vi "Auto Move Straight.vi"(6 "Target Angle":dbl, 7 "Target Distance":dbl=15.0 format="%#_13g", 8 "Error In":errorcluster, 11 "Refnum's In":T1) -> (0 "Error Out":errorcluster, 3 "Refnum's Out":T1)   [LabVIEW 2016]
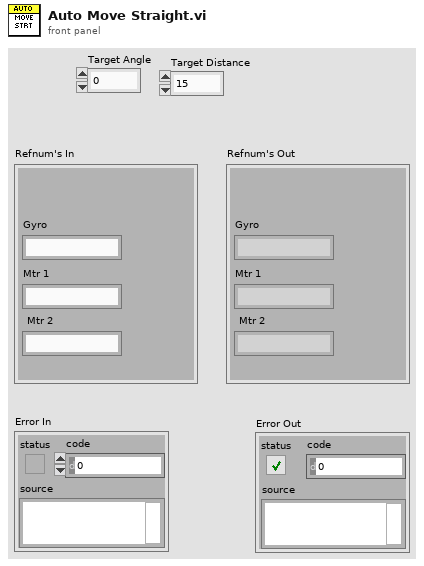
[diagram p1: front panel]
types:
  T1 = cluster{"Gyro":string, "Mtr 1":string, "Mtr 2":string}
  T2 = typedef "WPI_MotorControlDeviceRef.ctl" = cluster{"DeviceStatus":errorcluster, "Type":T3, "PWM":cluster{"PWM Channel":T4, "DeadBand":T5}, "CAN":cluster{"Device Number":u8, "SetOutput VI Ref":variant, "GetOutput VI Ref":variant, "Enable VI Ref":variant, "Disable VI Ref":variant, "Data":variant}, "Invert":bool}
  T3 = typedef "WPI_MotorControlType.ctl" = enum16{"PWM", "CAN"}
  T4 = typedef "FPGA_DIOPWMChannel.ctl" = enum8{"PWM 0", "PWM 1", "PWM 2", "PWM 3", "PWM 4", "PWM 5", "PWM 6", "PWM 7", "PWM 8", "PWM 9", "PWM MXP 0", "PWM MXP 1", "PWM MXP 2", "PWM MXP 3", "PWM MXP 4", "PWM MXP 5", "PWM MXP 6", "PWM MXP 7", "PWM MXP 8", "PWM MXP 9", "Invalid"}
  T5 = typedef "WPI_PWMDeadband.ctl" = cluster{"Name":string, "maxPositivePwm":i32, "minPositivePwm":i32, "centerPwm":i32, "maxNegativePwm":i32, "minNegativePwm":i32, "angularRange":u16}
  T6 = typedef "WPI_GyroDevRef.ctl" = cluster{"DevStatus":errorcluster, "Analog Channel":T7, "Offset":dbl, "Gain (VoltsPerDegree/Second)":dbl, "Gyro Type":enum16{"Analog", "XRS450"}, "Handle":i32, "SPI Bus":T8, "Device Found":bool, "Sample Rate":dbl, "Calibrate On Open":bool}
  T7 = typedef "FPGA_AIChannel.ctl" = enum8{"AI 0", "AI 1", "AI 2", "AI 3", "AI MXP 0", "AI MXP 1", "AI MXP 2", "AI MXP 3", "Invalid"}
  T8 = typedef "spi_bus.ctl" = enum16{"SPI On-Board, CS0", "SPI On-Board, CS1", "SPI On-Board, CS2", "SPI On-Board, CS3", "SPI MXP", "Invalid"}
  T9 = typedef "WPI_CANTalonSRX_GlobalStatus.ctl" = cluster{"Applied Throttle":dbl, "Module Enabled":bool, "CAN Error":errorcluster, "Closed Loop Error":dbl, "Forward Limit Switch Closed":bool, "Reverse Limit Switch Closed":bool, "Sensor Position":dbl, "Sensor Velocity":dbl, "Current":dbl, "Sticky Fault - Over Temp":bool, "Sticky Fault - Under Voltage":bool, "Sticky Fault - Forward Limit":bool, "Sticky Fault - Reverse Limit":bool, "Sticky Fault - Forward Soft Limit":bool, "Sticky Fault - Reverse Soft Limit":bool, "Brake is Enabled":bool, "Encoder Position":dbl, "Encoder Velocity":dbl, "Encoder Index Count":dbl, "Encoder A Pin State":bool, "Encoder B Pin State":bool, "Encoder Index Pin State":bool, "Analog In":dbl, "Analog In Velocity":dbl, "Temperature (C)":dbl, "Battery Voltage":dbl, "Control 5 Is Supported":bool, "Current Profile Slot Select":dbl, "Pos Div 8":bool, "Vel Div 4":bool, "Pulse Width Position":i32, "Pulse Width Velocity":i32, "Pulse Width Rise To Rise (us)":i32, "Pulse Width Rise To Fall (us)":i32, "Mot Prof Active Is Under Run":bool, "Mot Prof Active Has Under Run":bool, "Mot Prof Active Is Last":bool, "Mot Prof Active Velocity Only":bool, "Mot Prof Active Is Valid":bool, "Mot Prof Buffer Is Full":bool, "Mot Prof Active Profile Slot Select":i32, "Mot Prof NextID":i32, "Mot Prof Count":i32, "Mot Prof Active Velocity":dbl, "Mot Prof Active Position":dbl, "Mot Prof Output Enable":i32}
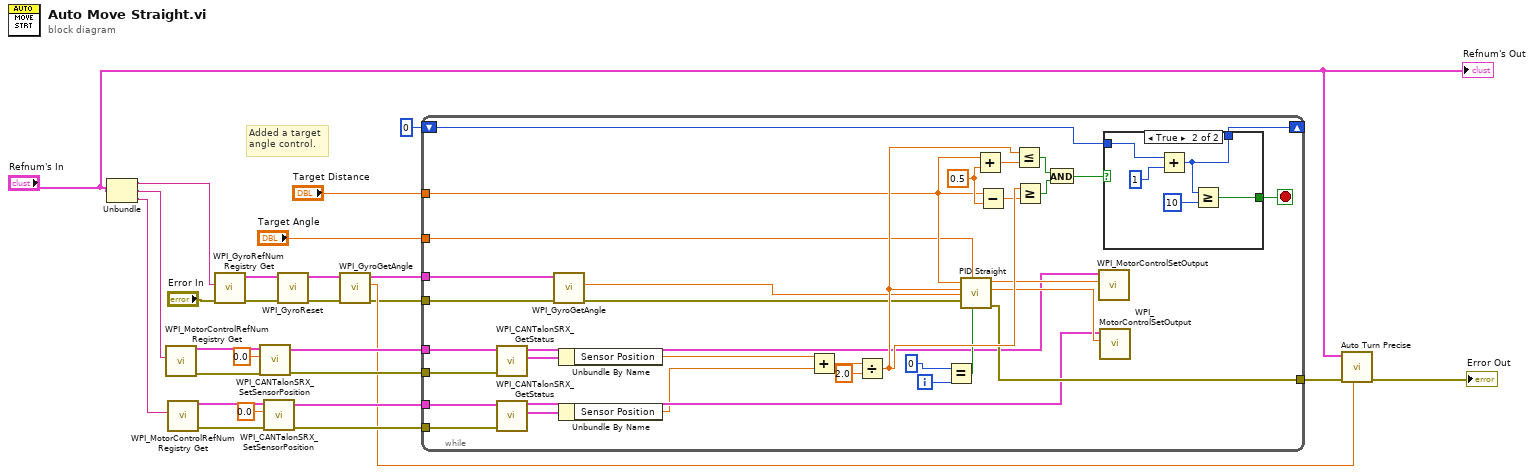
[diagram p0: block diagram]
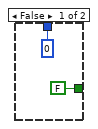
[diagram p2: hidden frame]
diagram:
  # "Added a target\nangle control."
  n1 = Unbundle("Refnum's In") -> ("Gyro"=w3:string, "Mtr 1"=w2:string, "Mtr 2"=w1:string)
  n2 = call <vilib>:"WPI_MotorControlRefNum Registry Get.vi"("refnum name"=w2) -> ("error out"=w15:errorcluster, "MotorControlDevRef"=w16:T2)  [unwired: 9 in]
  n3 = call <vilib>:"WPI_MotorControlRefNum Registry Get.vi"("refnum name"=w1) -> ("error out"=w20:errorcluster, "MotorControlDevRef"=w21:T2)  [unwired: 9 in]
  n4 = call <vilib>:"WPI_GyroRefNum Registry Get.vi"("error in (no error)"="Error In", "refnum name"=w3) -> ("error out"=w8:errorcluster, "GyroDevRef"=w7:T6)  [unwired: 8 in]
  n5 = call <vilib>:"WPI_CANTalonSRX_SetSensorPosition.vi"("error in (no error)"=w15, "New Sensor Position"=0.0, "CAN Talon SRX Ref"=w16) -> ("error out"=w14:errorcluster, "CAN Talon SRX Ref"=w13:T2)  [unwired: 7 in]
  n6 = call <vilib>:"WPI_CANTalonSRX_SetSensorPosition.vi"("error in (no error)"=w20, "New Sensor Position"=0.0, "CAN Talon SRX Ref"=w21) -> ("error out"=w19:errorcluster, "CAN Talon SRX Ref"=w18:T2)  [unwired: 7 in]
  n7 = call <vilib>:"WPI_GyroReset.vi"("error in"=w8, "GyroDevRef"=w7) -> ("error out"=w6:errorcluster, "GyroDevRef"=w5:T6)  [unwired: 8 in]
  n8 = call <vilib>:"WPI_GyroGetAngle.vi"("error in"=w6, "GyroDevRef"=w5) -> ("error out"=w10:errorcluster, "Angle"=w11:dbl, "GyroDevRef"=w9:T6)  [unwired: 5 in, 2 out]
  n9 = while {
    shift-right: [w48] -> _
    shift-left: 0 -> [w47]
    tunnel: "Target Distance" -> [w29]
    tunnel: [w43] -> w26
    tunnel: "Target Angle" -> [w28]
    tunnel: w9 -> [w35]
    tunnel: w10 -> [w34]
    tunnel: w19 -> [w33]
    tunnel: w18 -> [w32]
    tunnel: w14 -> [w31]
    tunnel: w13 -> [w30]
    i -> [w61]
    stop <- w42 stop-if-true
    w55 = 0.5 ("y")
    n10 = call <vilib>:"WPI_CANTalonSRX_GetStatus.vi"("error in (no error)"=w31, "CAN Talon SRX Ref"=w30) -> ("Talon SRX Status"=w56:T9, "CAN Talon SRX Ref"=w38:T2)  [unwired: 7 in, 1 out]
    n11 = call <vilib>:"WPI_CANTalonSRX_GetStatus.vi"("error in (no error)"=w33, "CAN Talon SRX Ref"=w32) -> ("Talon SRX Status"=w57:T9, "CAN Talon SRX Ref"=w39:T2)  [unwired: 7 in, 1 out]
    n12 = call <vilib>:"WPI_GyroGetAngle.vi"("error in"=w34, "GyroDevRef"=w35) -> ("error out"=w44:errorcluster, "Angle"=w46:dbl)  [unwired: 5 in, 3 out]
    n13 = Unbundle By Name(w56) -> ("Sensor Position"=w37:dbl)
    n14 = Unbundle By Name(w57) -> ("Sensor Position"=w36:dbl)
    n15 = Add(x=w37, y=w36) -> (x+y=w58:dbl)
    n16 = Divide(x=w58, y=2.0) -> (x/y=w53:dbl)
    n17 = Equal?(x=0, y=w61) -> (x = y?=w45:bool)
    n18 = call "PID Straight.vi"("Reinitialize"=w45, "Target Angle"=w28, "Error In"=w44, "Gyro Angle"=w46, "Current Distance"=w53, "Target Distance"=w29) -> ("Error Out"=w43:errorcluster, "Right Power"=w40:dbl, "Left Power"=w41:dbl)  [unwired: 3 in]
    n19 = Add(x=w29, y=w55) -> (x+y=w54:dbl)
    n20 = Subtract(x=w29, y=w55) -> (x-y=w52:dbl)
    n21 = Less Or Equal?(x=w53, y=w54) -> (x <= y?=w51:bool)
    n22 = Greater Or Equal?(x=w53, y=w52) -> (x >= y?=w50:bool)
    n23 = And(x=w51, y=w50) -> (x .and. y?=w49:bool)
    n24 = call <vilib>:"WPI_MotorControlSetOutput.vi"("Output"=w41, "MotorControlDevRef"=w38) -> ()  [unwired: 7 in, 3 out]
    n25 = call <vilib>:"WPI_MotorControlSetOutput.vi"("Output"=w40, "MotorControlDevRef"=w39) -> ()  [unwired: 7 in, 3 out]
    n26 = case shown="True" w49 {
      tunnel: w47 -> [_ w67]
      tunnel: [0 w66] -> w48
      tunnel: [FALSE w64] -> w42
      frame False {
      }
      frame True {
        n27 = Add(x=w67, y=1) -> (x+y=w66:i32)
        n28 = Greater Or Equal?(x=w66, y=10) -> (x >= y?=w64:bool)
      }
    }
  }
  n29 = call "Auto Turn Precise.vi"("Target Distance"=w11, "Error In"=w26, "Refnum's In"="Refnum's In") -> ("Error Out"=→"Error Out":errorcluster)  [unwired: 7 in, 1 out]
  "Refnum's Out" <- "Refnum's In"
